vi "HH_Test.vi"() -> ()   [LabVIEW 2011]
panel:
  out "Sync Rate":i32
  out "Range":i32
  out "Resolution (ps)":dbl
  out "error out":errorcluster
  out "Library Version":string="2.1"
  in  "error in (no error)":errorcluster
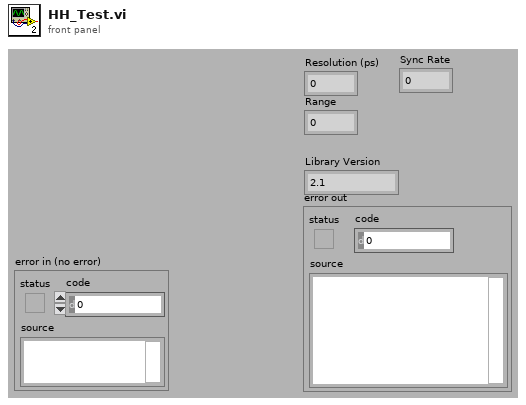
[diagram p1: front panel]
types:
  T1 = cluster{"Dev":i32, "SerNo":string, "HW_Model":string, "HW_Partno":string}[]
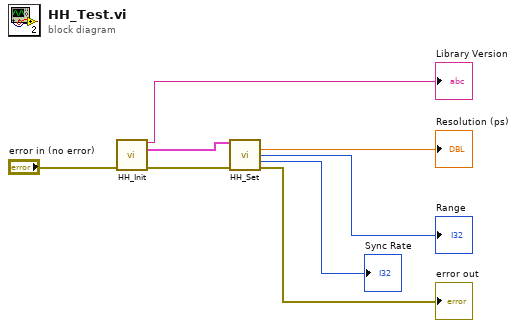
[diagram p0: block diagram]
diagram:
  n1 = call "HH_Init.vi"("error in (no error)"="error in (no error)") -> ("Library Version"=→"Library Version":string, "Device List"=w6:T1, "error out"=w7:errorcluster)  [unwired: 12 in]
  n2 = call "HH_Set.vi"("Device List"=w6, "error in (no error)"=w7) -> ("Resolution (ps)"=→"Resolution (ps)":dbl, "Range"=→"Range":i32, "Sync Rate"=→"Sync Rate":i32, "error out"=→"error out":errorcluster)  [unwired: 9 in, 1 out]
